vi "logging_set_split.vi"(7 "Evaluate section error (F)":bool, 8 "error in":errorcluster caption="error in (no error)", 11 "VISA resource name":refnum<visa-resource-name>) -> (0 "error out":errorcluster, 3 "VISA resource name out":refnum<visa-resource-name>)   [LabVIEW 2020, in "Rohde&Schwarz RTx Oscilloscopes.lvlib" / "rsidr_core.lvlib"]
uses:
  rsidr_core.lvlib
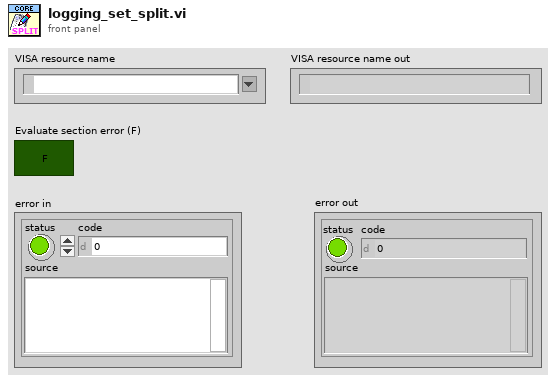
[diagram p1: front panel]
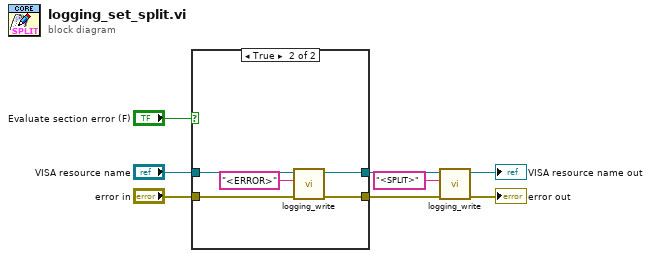
[diagram p0: block diagram]
diagram:
  n1 = case shown="True" "Evaluate section error (F)" {
    tunnel: "error in" -> [w10 w14]
    tunnel: "VISA resource name" -> [w9 w13]
    tunnel: [w10 w12] -> w2
    tunnel: [w9 w11] -> w1
    frame False {
    }
    frame True {
      n2 = call "logging_write.vi"("error in"=w14, "String to write"="<ERROR>", "VISA resource name"=w13) -> ("error out"=w12:errorcluster, "VISA resource name out"=w11:refnum<visa-resource-name>)  [unwired: 7 in]
    }
  }
  n3 = call "logging_write.vi"("error in"=w2, "String to write"="<SPLIT>", "VISA resource name"=w1) -> ("error out"=→"error out":errorcluster, "VISA resource name out"=→"VISA resource name out":refnum<visa-resource-name>)  [unwired: 7 in]
